vi "Initiate.vi"(8 "error in (no error)":errorcluster, 11 "VISA resource name":refnum<visa-resource-name>) -> (0 "error out":errorcluster, 3 "VISA resource name out":refnum<visa-resource-name>)   [LabVIEW 2012, in "RIGOL DS1000 Series.lvlib"]
doc: "Initiates a waveform acquisition.\n\n<B>Note:</B>\n Use this VI only with other low-level VIs."
uses:
  RIGOL DS1000 Series.lvlib
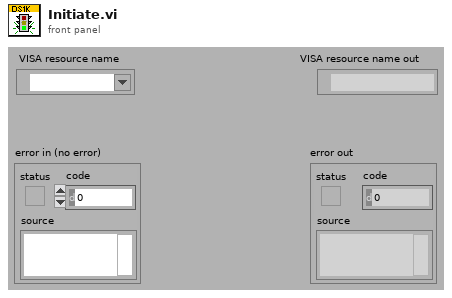
[diagram p1: front panel]
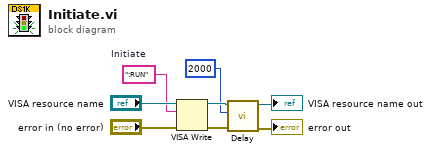
[diagram p0: block diagram]
diagram:
  w6 = ":RUN"  # Initiate
  n1 = VISA Write(VISA resource name="VISA resource name", write buffer=w6, error in (no error)="error in (no error)") -> (VISA resource name out=w5:refnum<visa-resource-name>, error out=w4:errorcluster)  [unwired: 1 out]
  n2 = call "Delay.vi"("error in (no error)"=w4, "Delay (ms)"=u32 2000, "VISA resource name"=w5) -> ("error out"=→"error out":errorcluster, "VISA resource name out"=→"VISA resource name out":refnum<visa-resource-name>)  [unwired: 7 out]
